vi "Get Interface.vi"(8 "error in (no error)":errorcluster, 11 "Output Actor in":refnum<class "Output Actor.lvclass">) -> (0 "error out":errorcluster, 2 "Output Actor Interface":refnum<class "Output Actor Interface.lvclass">, 3 "Output Actor out":refnum<class "Output Actor.lvclass">)   [LabVIEW 2015, in "Output Actor.lvclass"]
uses:
  Output Actor.lvclass
  Output Actor Interface/Output Actor Interface.lvclass
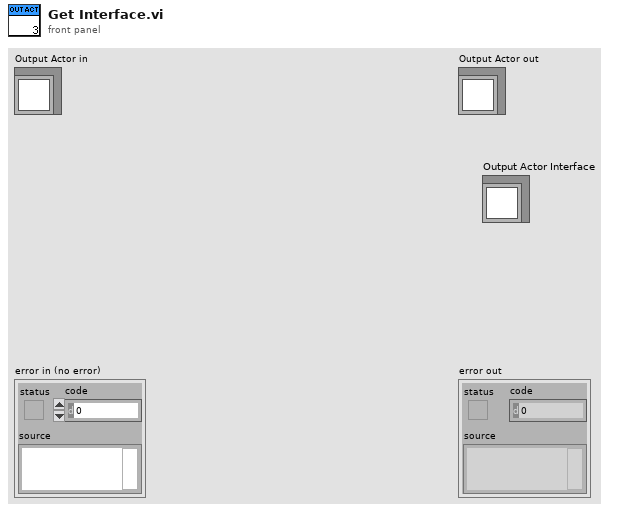
[diagram p1: front panel]
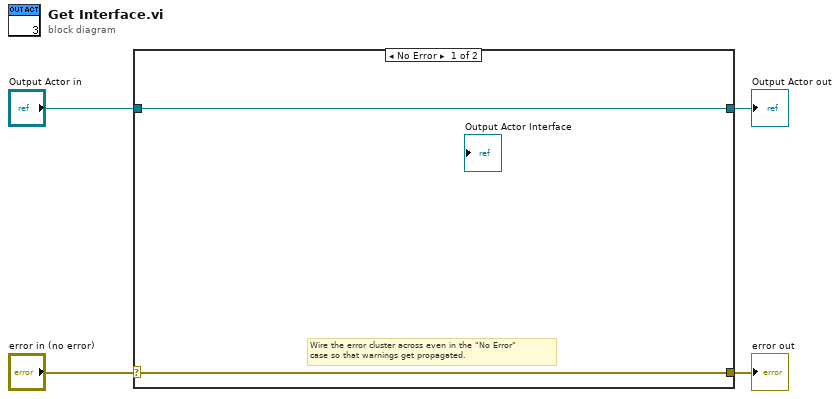
[diagram p0: block diagram]
diagram:
  n1 = case shown="No Error" "error in (no error)" {
    selector: "error in (no error)" -> [w5 w8]
    tunnel: [w5 w8] -> w3
    tunnel: [w6 w7] -> w1
    tunnel: "Output Actor in" -> [w6 w7]
    frame No Error {
      # "Wire the error cluster across even in the \"No Error\"\ncase so that warnings get propagated."
    }
    frame Error {
    }
  }
  "error out" <- w3
  "Output Actor out" <- w1
